vi "Save Data.vi"   [LabVIEW 2015]
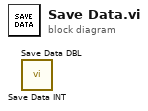
[diagram p0: block diagram]
diagram:
  n1 = call "Save Data INT.vi"() -> ()  [unwired: 10 in, 2 out]
  n2 = call "Save Data DBL.vi"() -> ()  [unwired: 10 in, 2 out]
